vi "ReadWebView.vi"(8 "Error In":errorcluster, 11 "object in":refnum<class "Component.lvclass">) -> (0 "Error Out":errorcluster, 2 "WebView":refnum<class "WebView2 Control.lvclass">, 3 "object out":refnum<class "Component.lvclass">)   [LabVIEW 2020, in "Component.lvclass"]
uses:
  Component.lvclass
  <vilib>/sklein/WebView2/Webview2 Lib/WebView2 Control Object/WebView2 Control.lvclass
  Component.lvclass/Component.ctl
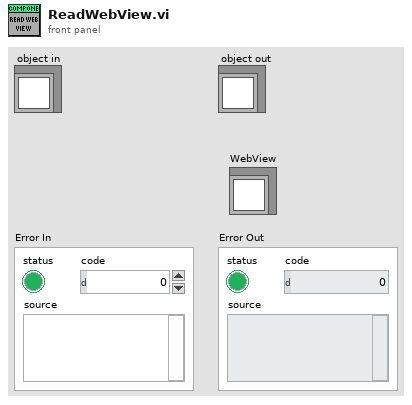
[diagram p1: front panel]
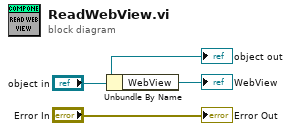
[diagram p0: block diagram]
diagram:
  n1 = Unbundle By Name("object in") -> ("WebView"=→"WebView":refnum<class "WebView2 Control.lvclass">)
  "Error Out" <- "Error In"
  "object out" <- "object in"
